vi "LINX - WS2812 Write N LEDs.vi"() -> ()   [LabVIEW 2019]
doc: "This example demonstrates how to set the color of a range of WS2812 LEDs."
uses:
  <vilib>/MakerHub/LINX/Public/Utilities/Open Serial.vi
  <vilib>/MakerHub/LINX/Public/Sensors/Lights/WS2812/Write N LEDs.vi
  <vilib>/MakerHub/LINX/LMH-LINX.lvlib
  <vilib>/MakerHub/LINX/Public/Sensors/Lights/WS2812/WS2812.lvlib
panel:
  in  "LED Colors":u32[](array[colorbox])=[16711680, 6618880, 16860]
  in  "LED Start Index":u16
  in  "Number of LEDs":u16=30
  in  "Data Channel":u8=11
  in  "Stop Button":bool
  in  "Serial Port":refnum<visa-resource-name>="COM6"
  # "WS2812 Write N LEDs Example\n\nThis example demonstrates how to set the color of a range of WS2812 LEDs.\n\nInstructions\n1. Select the COM Port associated with the LINX Device.\n2. Select the Data Channel and Number of LEDs.\n3. Click the Run Arrow.\n4. Select the index of the first LED to set.\n5. The number values in the color array determines how many LEDs will be set, starting with the LED at the LED Start Index."
  # "Set WS2812"
  # "LINX Device Settings"
  # "WS2812 Settings"
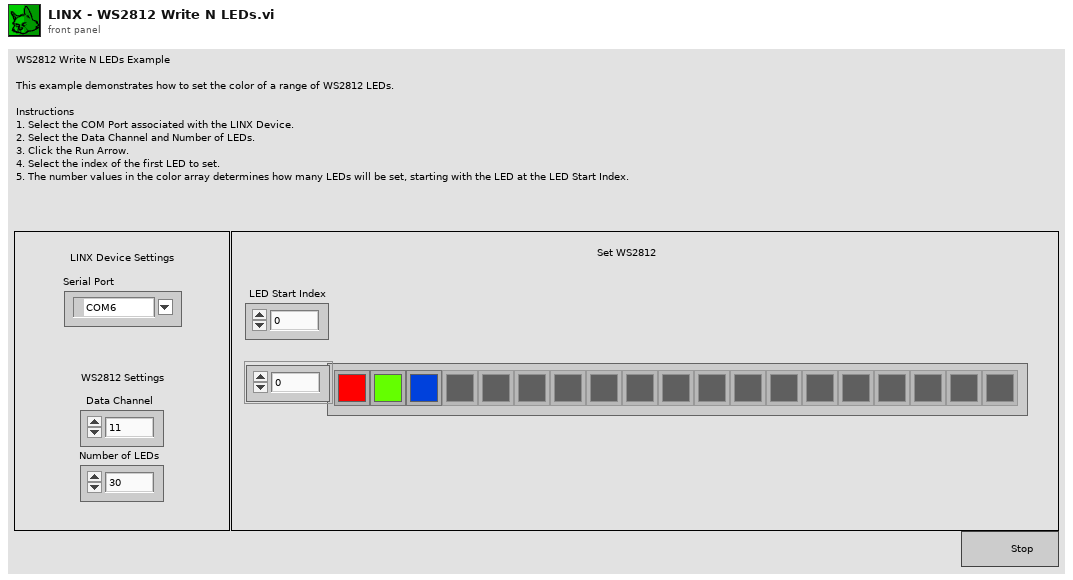
[diagram p1: front panel]
types:
  T1 = typedef "LMH-LINX.lvlib/LINX Ref.ctl" = cluster{"IO":T2, "Interface":T3, "LINX Device Config":T4}
  T2 = typedef "LMH-LINX.lvlib/Platform.ctl" = enum16{"Remote", "Local"}
  T3 = typedef "LMH-LINX.lvlib/Interface.ctl" = enum16{"Serial", "TCP"}
  T4 = typedef "LMH-LINX.lvlib/Device.lvlib/LINX Device Config.ctl" = cluster{"Interface":T3, "COM Port":refnum<visa-resource-name>, "TCP Configuration":T5, "Device Family":u8, "Device ID":u8, "Device Name":string, "TCP Ref":refnum<k5>, "Channels":T6}
  T5 = typedef "LMH-LINX.lvlib/Device.lvlib/TCP Config.ctl" = cluster{"IP Address":string, "Port":u16}
  T6 = typedef "LMH-LINX.lvlib/Channels.ctl" = cluster{"DI":u8[], "DO":u8[], "AI":u8[], "AO":u8[], "PWM":u8[], "QE":u8[], "UART":u8[], "I2C 2":u8[], "SPI":u8[], "CAN":u8[], "Servo":u8[], "AI Ref (V)":dbl, "AI Resolution (Bits)":u8, "AO Ref (V)":dbl, "AO Resolution (Bits)":u8}
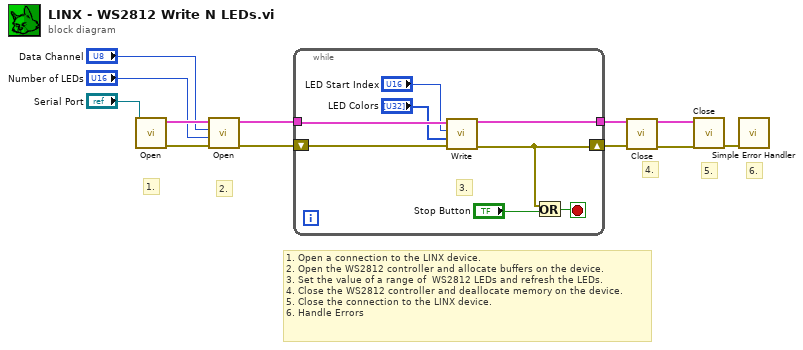
[diagram p0: block diagram]
diagram:
  # "4."
  # "2."
  # "1. Open a connection to the LINX device.\n2. Open the WS2812 controller and allocate buffers on the device.\n3. Set the value of a range of  WS2812 LEDs and refresh the LEDs.\n4. Close the WS2812 controller and deallocate memory on the device.\n5. Close the connection to the LINX device.\n6. Handle Errors"
  # "6."
  # "5."
  # "1."
  n1 = call-poly <vilib>:"Open.vi"("Serial Port"="Serial Port") -> ("Error Out"=w9:errorcluster, "LINX Resource"=w10:T1)  [unwired: 8 in, 1 out]
  n2 = call <vilib>:"Open.vi"("Error In"=w9, "Number of LEDs"="Number of LEDs", "Data Channel"="Data Channel", "LINX Resource"=w10) -> ("Error Out"=w8:errorcluster, "LINX Resource"=w7:T1)  [unwired: 6 in]
  n3 = while {
    tunnel: w7 -> [w17]
    shift-right: [w14] -> w4
    shift-left: w8 -> [w18]
    tunnel: [w15] -> w3
    stop <- w20 stop-if-true
    # "3."
    n4 = call-poly <vilib>:"Write.vi"("Error In"=w18, "Colors"="LED Colors", "LED Index"="LED Start Index", "LINX Ref"=w17) -> ("Error Out"=w14:errorcluster, "LINX Ref"=w15:T1)  [unwired: 6 in]
    n5 = Or(x=w14, y="Stop Button") -> (x .or. y?=w20:bool)
  }
  n6 = call <vilib>:"Close.vi"("Error In"=w4, "LINX Resource"=w3) -> ("Error Out"=w2:errorcluster, "LINX Resource"=w1:T1)  [unwired: 8 in]
  n7 = call <vilib>:"Close.vi"("Error In"=w2, "LINX Resource"=w1) -> ("Error Out"=w11:errorcluster)  [unwired: 9 in]
  n8 = call <vilib>:"Simple Error Handler.vi"("error in (no error)"=w11) -> ()  [unwired: 4 in, 5 out]
